vi "createScriptEvent.vi"(8 "error in (no error)":errorcluster, 10 "action":T1(ring)) -> (0 "error out":errorcluster, 3 "ScriptEvent out":refnum<class "ScriptEvent.lvclass">)   [LabVIEW 2009, in "Tools.lvlib" / "Scripting.lvlib" / "ScriptEvent.lvclass"]
uses:
  ScriptEvent.lvclass
  Ramp/RampEvent/RampEvent.lvclass
  SingleTone/SingleTone.lvclass
  SingleTone/SingleToneRamp/SingleToneRamp.lvclass
  Rf Event/rf.lvclass
  RfRamp/RfRamp.lvclass
  Delay/Delay.lvclass
  ScriptEvent.lvclass/ScriptEvent.ctl
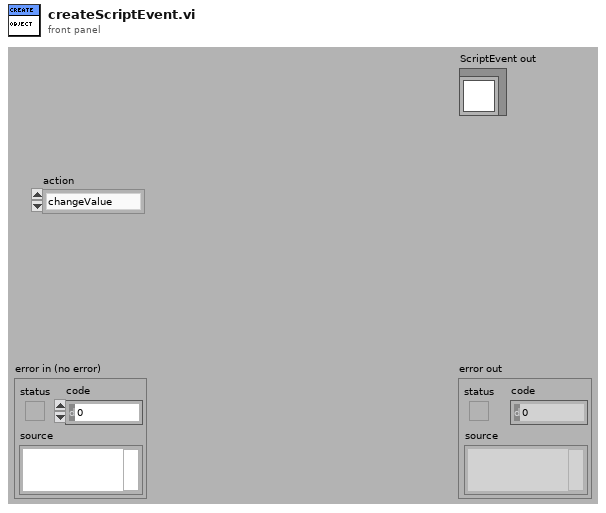
[diagram p1: front panel]
types:
  T1 = enum16{"changeValue", "pulse", "clock", "rampUp", "rampDown", "singleTone", "singleToneRamp", "playFile", "rf", "rfRamp", "delay"}
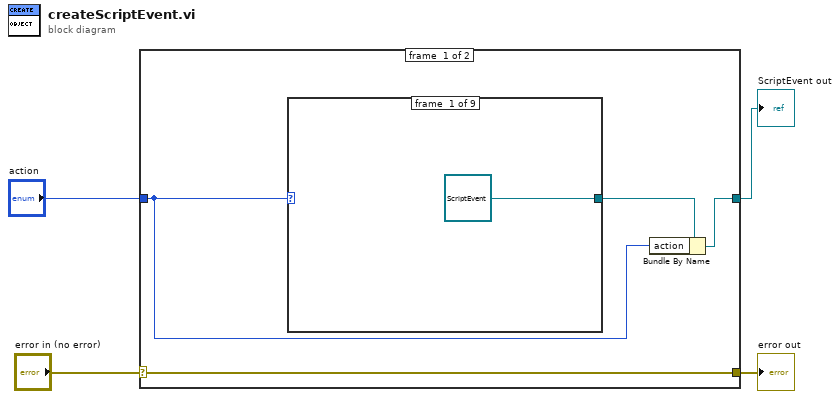
[diagram p0: block diagram]
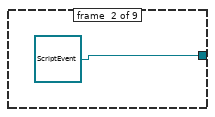
[diagram p2: hidden frame]
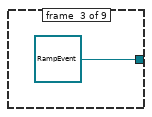
[diagram p3: hidden frame]
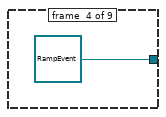
[diagram p4: hidden frame]
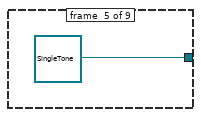
[diagram p5: hidden frame]
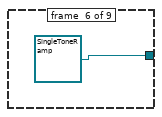
[diagram p6: hidden frame]
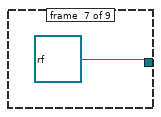
[diagram p7: hidden frame]
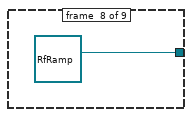
[diagram p8: hidden frame]
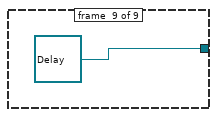
[diagram p9: hidden frame]
diagram:
  n1 = case shown="No Error" "error in (no error)" {
    selector: "error in (no error)" -> [w8 w18]
    tunnel: [w8 w18] -> w3
    tunnel: "action" -> [w5 _]
    tunnel: [w7 _] -> w1
    frame #0 {
      n2 = case shown="\"delay\"" w5 {
        tunnel: [refnum<class "ScriptEvent.lvclass"> refnum ("Tools.lvlib:Scripting.lvlib:ScriptEvent.lvclass") refnum<class "ScriptEvent.lvclass"> refnum ("Tools.lvlib:Scripting.lvlib:ScriptEvent.lvclass") refnum<class "RampEvent.lvclass"> refnum ("Tools.lvlib:Scripting.lvlib:RampEvent.lvclass") refnum<class "RampEvent.lvclass"> refnum ("Tools.lvlib:Scripting.lvlib:RampEvent.lvclass") refnum<class "SingleTone.lvclass"> refnum ("Tools.lvlib:Scripting.lvlib:SingleTone.lvclass") refnum<class "SingleToneRamp.lvclass"> refnum ("Tools.lvlib:Scripting.lvlib:SingleToneRamp.lvclass") refnum<class "rf.lvclass"> refnum ("Tools.lvlib:Scripting.lvlib:rf.lvclass") refnum<class "RfRamp.lvclass"> refnum ("Tools.lvlib:Scripting.lvlib:RfRamp.lvclass") refnum<class "Delay.lvclass"> refnum ("Tools.lvlib:Scripting.lvlib:Delay.lvclass")] -> w6
        frame #0 {
        }
        frame #1 {
        }
        frame #2 {
        }
        frame #3 {
        }
        frame #4 {
        }
        frame #5 {
        }
        frame #6 {
        }
        frame #7 {
        }
        frame #8 {
        }
      }
      n3 = Bundle By Name(cluster=w6, "action"=w5) -> (w7:refnum<class "ScriptEvent.lvclass">)
    }
    frame #1 {
    }
  }
  "error out" <- w3
  "ScriptEvent out" <- w1
